vi "Evaluate Part 1.vi"() -> ()   [LabVIEW 2020]
uses:
  Card/Card.lvclass
panel:
  out "sum":i32=13
  in  "Input":string="Card 1: 41 48 83 86 17 | 83 86  6 31 17  9 48 53\nCard 2: 13 32 20 16 61 | 61 30 68 82 17 32 24 19\nCard 3:  1 21 53 59 44 | 69 82 63 72 16 21 14  1\nCard 4: 41 92 73 84 69 | 59 84 76 51 58  5 54 83\nCard 5: 87 83 26 28 32 | 88 30 70 12 93 22 82 36\nCard 6: 31 18 13 56 72 | 74 77 10 23 35 67 36 11"
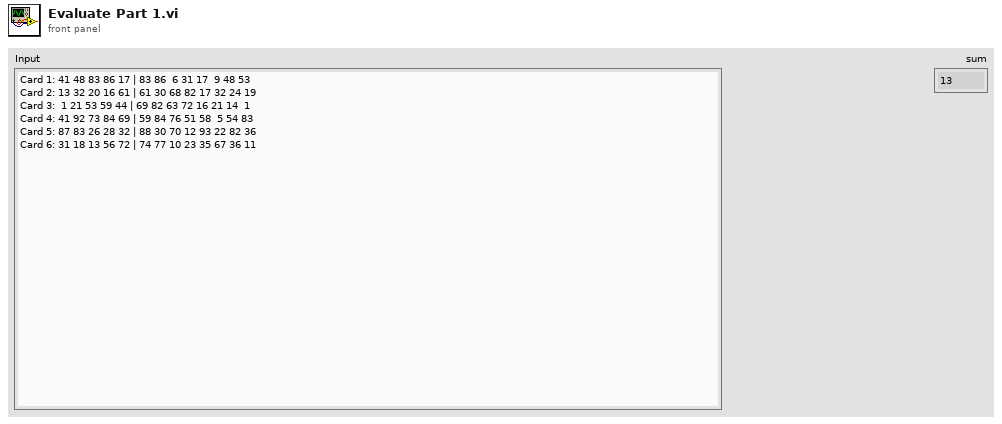
[diagram p1: front panel]
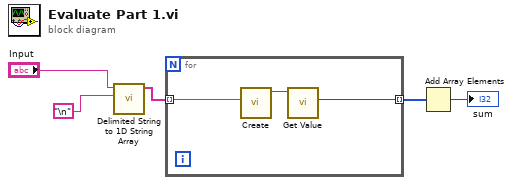
[diagram p0: block diagram]
diagram:
  n1 = call <vilib>:"Delimited String to 1D String Array.vi"("delimiter"="\n", "delimited string"="Input") -> ("string array"=w3:string[])  [unwired: 9 in]
  n2 = for {
    tunnel: w3 -> [w8] mode=indexing
    tunnel: [w6] -> w2 mode=indexing
    n3 = call "Create.vi"("Card"=w8) -> ("Card"=w7:refnum<class "Card.lvclass">)  [unwired: 9 in, 1 out]
    n4 = call-dynamic "Get Value.vi"("Card in"=w7) -> ("Value"=w6:i32)  [unwired: 8 in, 2 out]
  }
  n5 = Add Array Elements(numeric array=w2) -> (sum=→"sum":i32)
